vi "Status_update_VS.vi"(8 "error in (no error)":errorcluster, 10 "Data Value Reference in":T4, 11 "Status_Cluster_out in":T1) -> (0 "error out":errorcluster, 3 "Status_Cluster_out out":T1)   [LabVIEW 2020, in "Vires VTD Engine.lvlib"]
doc: "Reads Connection Command from VS, makes case selection for next iteration and writes status update to VS."
uses:
  Vires VTD Engine.lvlib
  Type/Status_Cluster.ctl
  Type/ConnectionStatus.ctl
  Type/CaseSelection.ctl
  <vilib>/NI/NIVS Inline Async API/_Data Access Engine/Data Access Engine/Types/ReadWrite.DVR.ctl
  <vilib>/NI/NIVS Inline Async API/_Data Access Engine/Access Type Classes/ReadWrite/ReadWrite.lvclass
  <vilib>/NI/NIVS Inline Async API/_Data Access Engine/Data Access Engine/Data Access Engine.lvclass
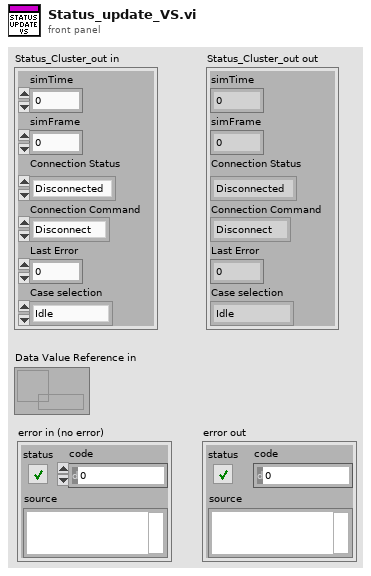
[diagram p1: front panel]
types:
  T1 = typedef "Vires VTD Engine.lvlib/Status_Cluster.ctl" = cluster{"simTime":dbl, "simFrame":dbl, "Connection Status":T2, "Connection Command":enum16{"Disconnect", "Connect"}, "Last Error":i32, "Case selection":T3}
  T2 = typedef "Vires VTD Engine.lvlib/ConnectionStatus.ctl" = enum16{"Disconnected", "Connected"}
  T3 = typedef "Vires VTD Engine.lvlib/CaseSelection.ctl" = enum32{"Idle", "Connecting", "Disconnecting", "Read/Write"}
  T4 = typedef "Data Access Engine.lvlib/Data Access Engine.lvclass/ReadWrite.DVR.ctl" = refnum<data-value>
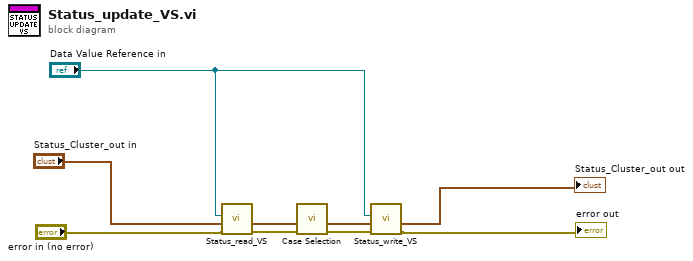
[diagram p0: block diagram]
diagram:
  n1 = call "Status_read_VS.vi"("error_in"="error in (no error)", "Status_Cluster_in"="Status_Cluster_out in", "Ref"="Data Value Reference in") -> ("error_out"=w2:errorcluster, "Status_Cluster_out"=w8:T1)  [unwired: 7 in]
  n2 = call "Case Selection.vi"("error in (no error)"=w2, "Status_Cluster_in"=w8) -> ("error out"=w4:errorcluster, "Status_Cluster_out"=w9:T1)  [unwired: 8 in]
  n3 = call "Status_write_VS.vi"("error_in"=w4, "Status_Cluster_in"=w9, "Ref"="Data Value Reference in") -> ("error_out"=→"error out":errorcluster, "Status_Cluster_out"=→"Status_Cluster_out out":T1)  [unwired: 7 in]
